vi "ConvertParameters.vi"(1 "filenames":path[](array[path])=[path "C:/CuspControl/GPIB and Network/Cusp/HVpulser.txt"]) -> (0 "Clusters Out":T1=[{"ao line"="ao0", "Duration, Gain, NewVal"=[0.0, 0.0]}, {"ao line"="ao1", "Duration, Gain, NewVal"=[0.0, 0.0]}, {"ao line"="ao2", "Duration, Gain, NewVal"=[0.0, 0.0]}] {"Duration, Gain, NewVal" format="%#_3g"})   [LabVIEW 2018]
uses:
  ParameterSubCluster.ctl
panel:
  out "array":string[][](array[string])=[["ao0", "0.000000E+0", "0.000000E+0"], ["ao1", "0.000000E+0", "0.000000E+0"], ["ao2", "0.000000E+0", "0.000000E+0"]]
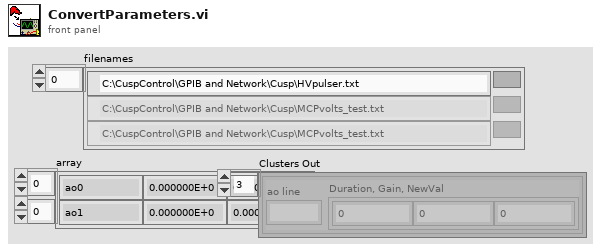
[diagram p1: front panel]
types:
  T1 = typedef "ParameterSubCluster.ctl" = cluster{"ao line":string, "Duration, Gain, NewVal":dbl[]}[]
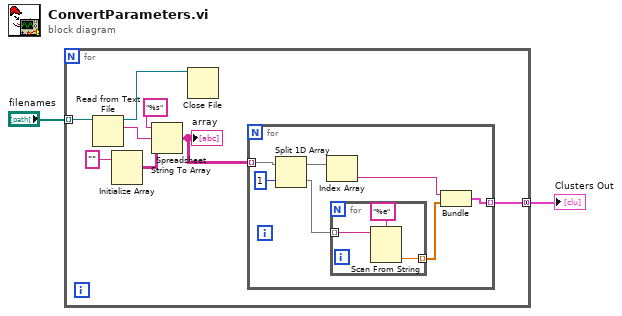
[diagram p0: block diagram]
diagram:
  n1 = for {
    tunnel: [w5] -> w2 mode=concatenating
    tunnel: "filenames" -> [w4] mode=indexing
    n2 = Read from Text File(file (use dialog)=w4) -> (refnum out=w10:refnum<file>, text=w9:string)  [unwired: 3 in, 2 out]
    n3 = Initialize Array("") -> (w7:string[][])  [unwired: 2 in]
    n4 = Spreadsheet String To Array(format string="%s", spreadsheet string=w9, array type (2D Dbl)=w7) -> (array=w3:string[][])  [unwired: 1 in]
    "array" <- w3
    n5 = Close File(refnum=w10) -> ()  [unwired: 1 in, 2 out]
    n6 = for {
      tunnel: w3 -> [w17] mode=indexing
      tunnel: [w12] -> w5 mode=indexing
      n7 = Split 1D Array(array=w17, index=1) -> (first subarray=w15:string[], second subarray=w14:string[])
      n8 = Index Array(array=w15) -> (element=w13:string)  [unwired: 1 in]
      n9 = for {
        tunnel: w14 -> [w20] mode=indexing
        tunnel: [w18] -> w11 mode=indexing
        n10 = Scan From String(format string="%e", input string=w20) -> (output 1=w18:dbl)  [unwired: 3 in, 3 out]
      }
      n11 = Bundle(w13, w11) -> (w12:cluster{string, dbl[]})  [unwired: 1 in]
    }
  }
  "Clusters Out" <- w2
